vi "MaxPool.vi"(9 "Convolution Settings":T1={"Stride"=3, "Offset - x"=0, "Offset - y"=0, "Round Up"=FALSE}, 10 "Pool Size":cluster{"X Size":i32, "Y Size":i32}, 11 "Data In":dbl[][][](array[numeric])) -> (3 "Data Out":dbl[][][](array[numeric]))   [LabVIEW 2018]
panel:
  out "Data After Buffer":dbl[][][](array[numeric])
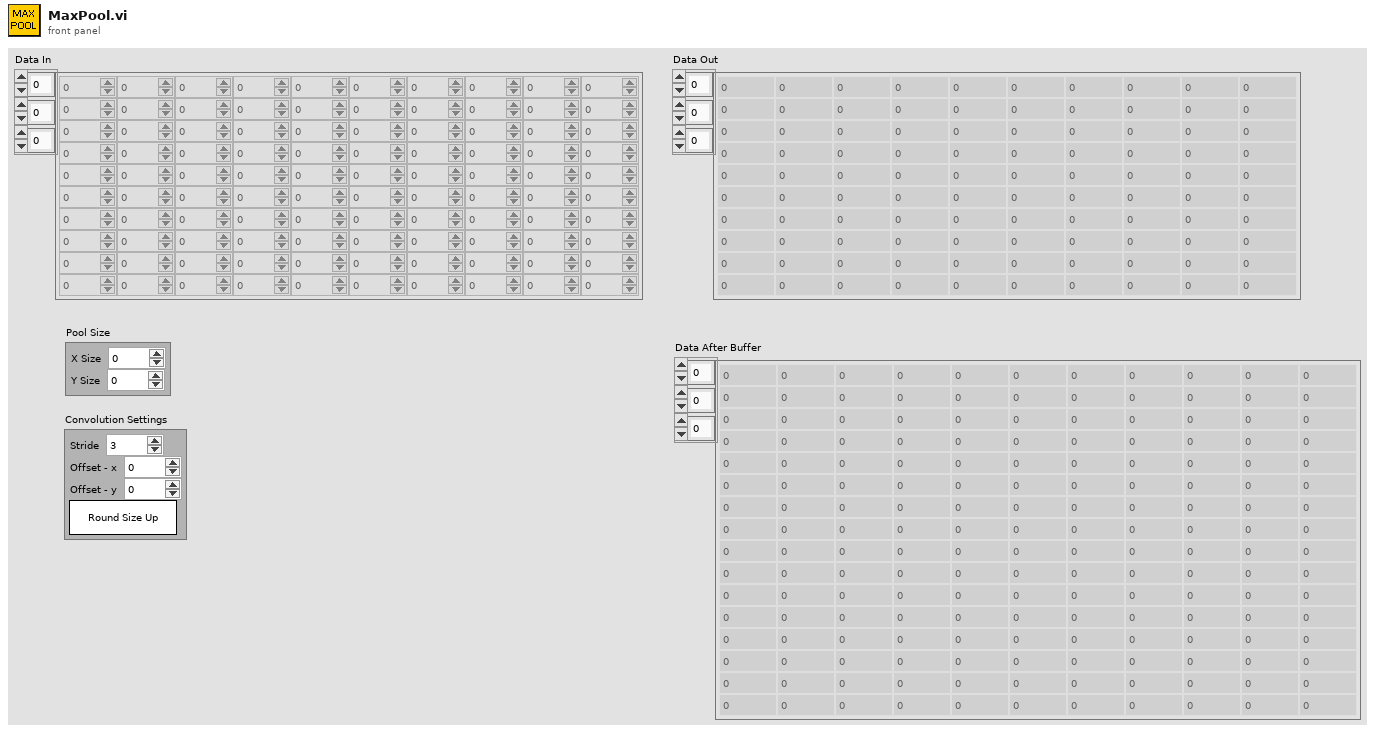
[diagram p1: front panel]
types:
  T1 = cluster{"Stride":i32, "Offset - x":i32, "Offset - y":i32, "Round Up":bool}
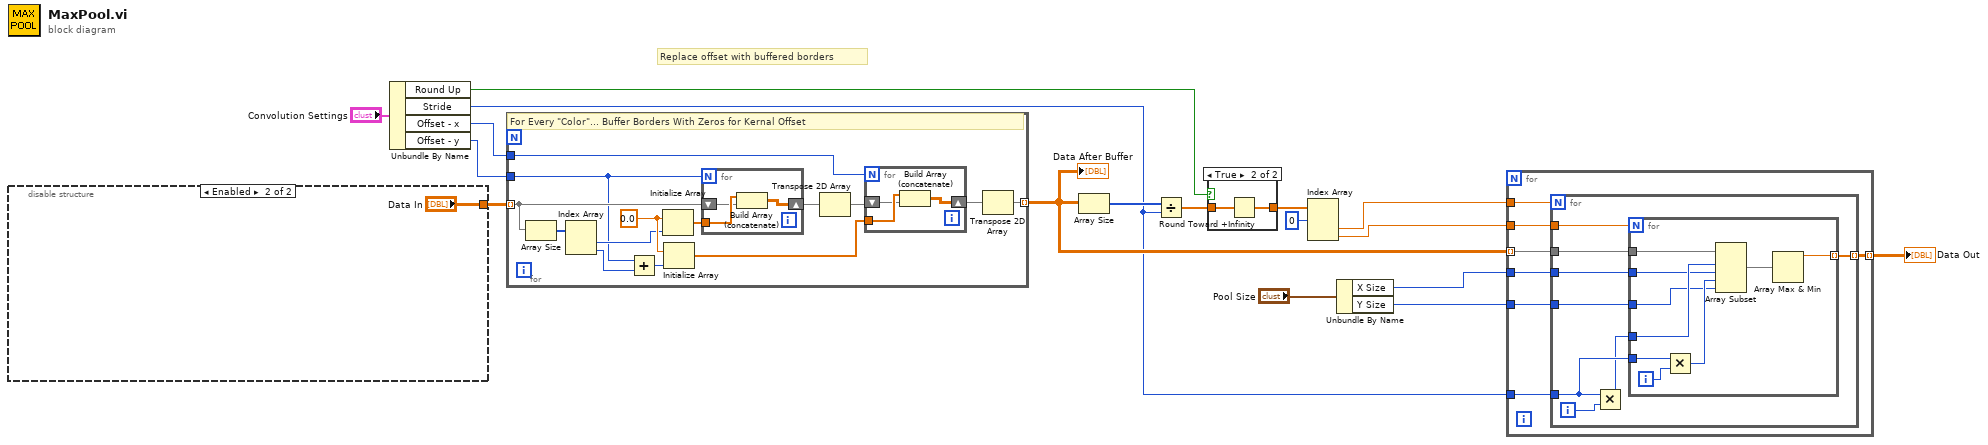
[diagram p0: block diagram]
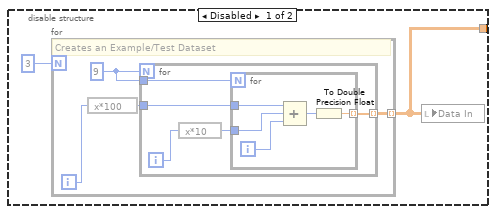
[diagram p2: hidden frame]
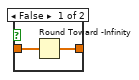
[diagram p3: hidden frame]
diagram:
  # "Replace offset with buffered borders"
  n1 = disable-structure shown="Enabled" {
    disable-tunnel: [w18 "Data In"] -> w9
    frame Disabled {
      n2 = for {
        N: 3 -> [_]
        tunnel: [w20] -> w18 mode=indexing
        i -> [w22]
        w23 = 9
        # "Creates an Example/Test Dataset"
        n3 = expression code="x*100"(w22) -> (w21:i32)
        n4 = for {
          N: w23 -> [_]
          tunnel: w23 -> [w28]
          tunnel: w21 -> [w27]
          tunnel: [w24] -> w20 mode=indexing
          i -> [w26]
          n5 = expression code="x*10"(w26) -> (w25:i32)
          n6 = for {
            N: w28 -> [_]
            tunnel: w27 -> [w31]
            tunnel: w25 -> [w33]
            tunnel: [w29] -> w24 mode=indexing
            i -> [w32]
            n7 = Compound Arithmetic op=ADD(w31, w33, w32) -> (w30:i32)
            n8 = To Double Precision Float(number=w30) -> (double precision float=w29:dbl)
          }
        }
      }
      n9 = local write "Data In"(w18) -> ()
    }
    frame Enabled {
    }
  }
  n10 = Unbundle By Name("Convolution Settings") -> ("Round Up"=w4:bool, "Stride"=w5:i32, "Offset - x"=w7:i32, "Offset - y"=w6:i32)
  n11 = for {
    tunnel: w6 -> [w35]
    tunnel: w9 -> [w42] mode=indexing
    tunnel: [w40] -> w12 mode=indexing
    tunnel: w7 -> [w37]
    w47 = 0.0 ("element")
    # "For Every \"Color\"... Buffer Borders With Zeros for Kernal Offset"
    n12 = Array Size(array=w42) -> (size(s)=w48:i32[])
    n13 = Index Array(array=w48) -> (element #1=w45:i32, element #2=w46:i32)  [unwired: 2 in]
    n14 = Add(x=w35, y=w46) -> (x+y=w44:i32)
    n15 = Initialize Array(w47, w45) -> (w43:dbl[])
    n16 = Initialize Array(w47, w44) -> (w38:dbl[])
    n17 = for {
      N: w35 -> [_]
      tunnel: w43 -> [w54]
      shift-right: [w52] -> w41
      shift-left: w42 -> [w53]
      n18 = Build Array (concatenate)(w54, w53) -> (w52:dbl[][])
    }
    n19 = Transpose 2D Array(2D array=w41) -> (transposed array=w39:dbl[][])
    n20 = for {
      N: w37 -> [_]
      tunnel: w38 -> [w51]
      shift-right: [w49] -> w36
      shift-left: w39 -> [w50]
      n21 = Build Array (concatenate)(w51, w50) -> (w49:dbl[][])
    }
    n22 = Transpose 2D Array(2D array=w36) -> (transposed array=w40:dbl[][])
  }
  "Data After Buffer" <- w12
  n23 = Array Size(array=w12) -> (size(s)=w13:i32[])
  n24 = Divide(x=w13, y=w5) -> (x/y=w14:dbl[])
  n25 = case shown="True" w4 {
    tunnel: [w55 w58] -> w15
    tunnel: w14 -> [w56 w57]
    frame False {
      n26 = Round Toward -Infinity(1:w56) -> (0:w55:dbl[])
    }
    frame True {
      n27 = Round Toward +Infinity(x=w57) -> (ceil(x): smallest int >= x=w58:dbl[])
    }
  }
  n28 = Index Array(array=w15, index #1=0 ("index")) -> (element #2=w11:dbl, element #3=w10:dbl)  [unwired: 2 in, 1 out]
  n29 = Unbundle By Name("Pool Size") -> ("X Size"=w2:i32, "Y Size"=w1:i32)
  n30 = for {
    tunnel: [w65] -> w17 mode=indexing
    tunnel: w12 -> [w64] mode=indexing
    tunnel: w11 -> [w63]
    tunnel: w10 -> [w62]
    tunnel: w5 -> [w61]
    tunnel: w2 -> [w60]
    tunnel: w1 -> [w59]
    n31 = for {
      N: w63 -> [_]
      tunnel: w62 -> [w73]
      tunnel: w61 -> [w71]
      tunnel: w64 -> [w69]
      tunnel: [w68] -> w65 mode=indexing
      tunnel: w60 -> [w67]
      tunnel: w59 -> [w66]
      i -> [w72]
      n32 = Multiply(x=w71, y=w72) -> (x*y=w70:i32)
      n33 = for {
        N: w73 -> [_]
        tunnel: w71 -> [w81]
        tunnel: w70 -> [w78]
        tunnel: w69 -> [w74]
        tunnel: [w79] -> w68 mode=indexing
        tunnel: w67 -> [w77]
        tunnel: w66 -> [w75]
        i -> [w82]
        n34 = Multiply(x=w81, y=w82) -> (x*y=w76:i32)
        n35 = Array Subset(array=w74, index (row)=w78, length (row)=w77, index (col)=w76, length (col)=w75) -> (w80:dbl[][])
        n36 = Array Max & Min(array=w80) -> (max value=w79:dbl)  [unwired: 3 out]
      }
    }
  }
  "Data Out" <- w17
